vi "RSNRPZ Initialize.vi"(8 "error in (no error)":errorcluster, 9 "Reset Device (T: Reset Device)":bool=TRUE, 10 "ID Query (T: Do Query)":bool=TRUE, 11 "Resource Name (USB::0x0aad::0x000b::100000)":string="USB::0x0aad::0x000b::100000") -> (0 "error out":errorcluster, 3 "dup VISA session":refnum<visa-resource-name>)   [LabVIEW 2019]
doc: "This VI performs the following initialization actions and assigned specified sesnor to channel 1:\n\n- Opens a session to the specified device using the interface and address specified in the Resource Name control.\n\n- Performs an identification query on the sensor.\n\n- Resets the instrument to a known state.\n\n- Sends initialization commands to the sensor\n\n- Returns an Instrument Handle which is used to differentiate between different sessions of this instrument driver."
uses:
  rsnrpz_32.dll
panel:
  # "Warning: The driver requires NRP Toolkit installed on your computer"
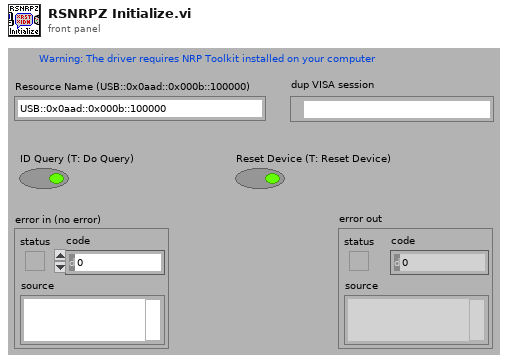
[diagram p1: front panel]
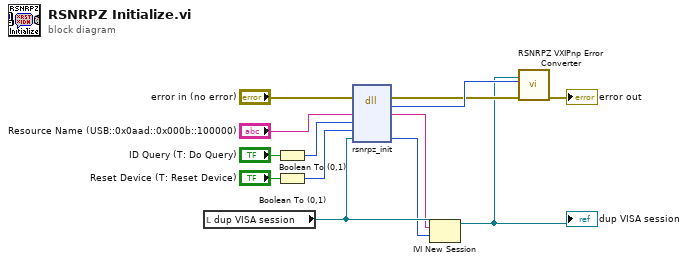
[diagram p0: block diagram]
diagram:
  n1 = local read "dup VISA session"() -> (w9:refnum<visa-resource-name>)
  n2 = Boolean To (0,1)(Boolean="ID Query (T: Do Query)") -> (0, 1=w6:i16)
  n3 = Boolean To (0,1)(Boolean="Reset Device (T: Reset Device)") -> (0, 1=w10:i16)
  n4 = dll-call lib="C:/Users/LABadmin/Documents/Jarvis/user_lib/rsnrpz/rsnrpz_32.dll" fn="rsnrpz_init"(error in="error in (no error)", "resourceName"="Resource Name (USB::0x0aad::0x000b::100000)", "IDQuery"=w6, "resetDevice"=w10, "instrumentHandle"=w9) -> (error out=w3:errorcluster, "return type"=w11:i32, "resourceName"=w8:string, "instrumentHandle"=w7:i32)  [unwired: 4 in, 1 out]
  n5 = IVI New Session(9:w7, 10:w8, 11:w9) -> (3:w1:refnum<visa-resource-name>)
  "dup VISA session" <- w1
  n6 = call <instrlib>:"RSNRPZ VXIPnp Error Converter.vi"("error in"=w3, "VXIPnp error code"=w11, "VISA session"=w1) -> ("error out"=→"error out":errorcluster)  [unwired: 7 in, 1 out]
